vi "VALEW_ATC_Get ATC Data.vi"(0 "GEA2 Reference In":refnum<k24>, 11 "Error In":errorcluster) -> (4 "GEA2 Reference Out":refnum<k24>, 8 "ATC Data":T1, 15 "Error Out":errorcluster)   [LabVIEW 2016, in "TLMB.lvlib"]
uses:
  Projects/TLMB.lvlib
  typedefs/VALEW_ATC_Data.ctl
  Q:/Common/DLLs/GEA3/GeaCommunication.dll
  Common/DLLs/GEA3/GeaCommunication.dll
  Common/LabVIEW GEA2 Toolkit/LabVIEW_GEA2_Toolkit.lvlibp/type defs/ERD Read Data In.ctl
  Common/LabVIEW GEA2 Toolkit/LabVIEW_GEA2_Toolkit.lvlibp/type defs/Data Type.ctl
  Common/LabVIEW GEA2 Toolkit/LabVIEW_GEA2_Toolkit.lvlibp/type defs/Source_Destination.ctl
  Common/LabVIEW GEA2 Toolkit/LabVIEW_GEA2_Toolkit.lvlibp
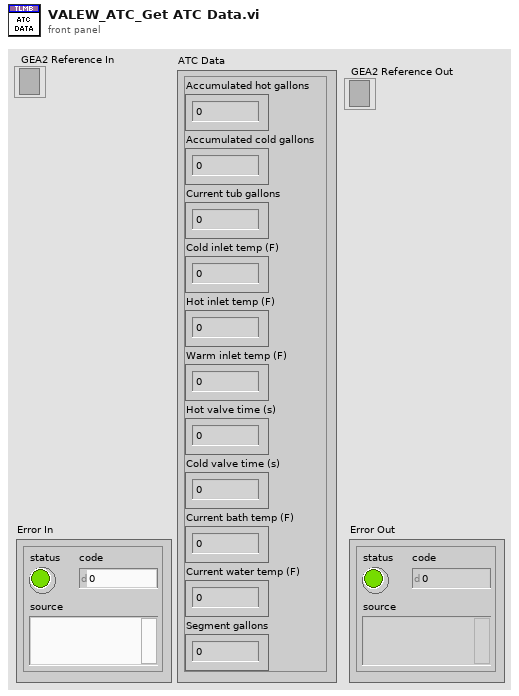
[diagram p1: front panel]
types:
  T1 = typedef "TLMB.lvlib/VALEW_ATC_Data.ctl" = cluster{"Accumulated hot gallons":dbl, "Accumulated cold gallons":dbl, "Current tub gallons":dbl, "Cold inlet temp (F)":dbl, "Hot inlet temp (F)":dbl, "Warm inlet temp (F)":dbl, "Hot valve time (s)":u16, "Cold valve time (s)":u16, "Current bath temp (F)":dbl, "Current water temp (F)":dbl, "Segment gallons":dbl}
  T2 = typedef "LabVIEW_GEA2_Toolkit.lvlibp/Source_Destination.ctl" = cluster{"Source":u8, "Destination":u8}
  T3 = typedef "LabVIEW_GEA2_Toolkit.lvlibp/ERD Read Data In.ctl" = cluster{"ERD Number":u16, "Data Type":T4}
  T4 = typedef "LabVIEW_GEA2_Toolkit.lvlibp/Data Type.ctl" = enum16{"string", "boolean", "uint8_t", "uint16_t", "uint32_t", "uint64_t", "int8_t", "int16_t", "int32_t", "int64_t"}
  T5 = typedef "LabVIEW_GEA2_Toolkit.lvlibp/ERD Read Data Out.ctl" = cluster{"ERD Number":u16, "Data":string}
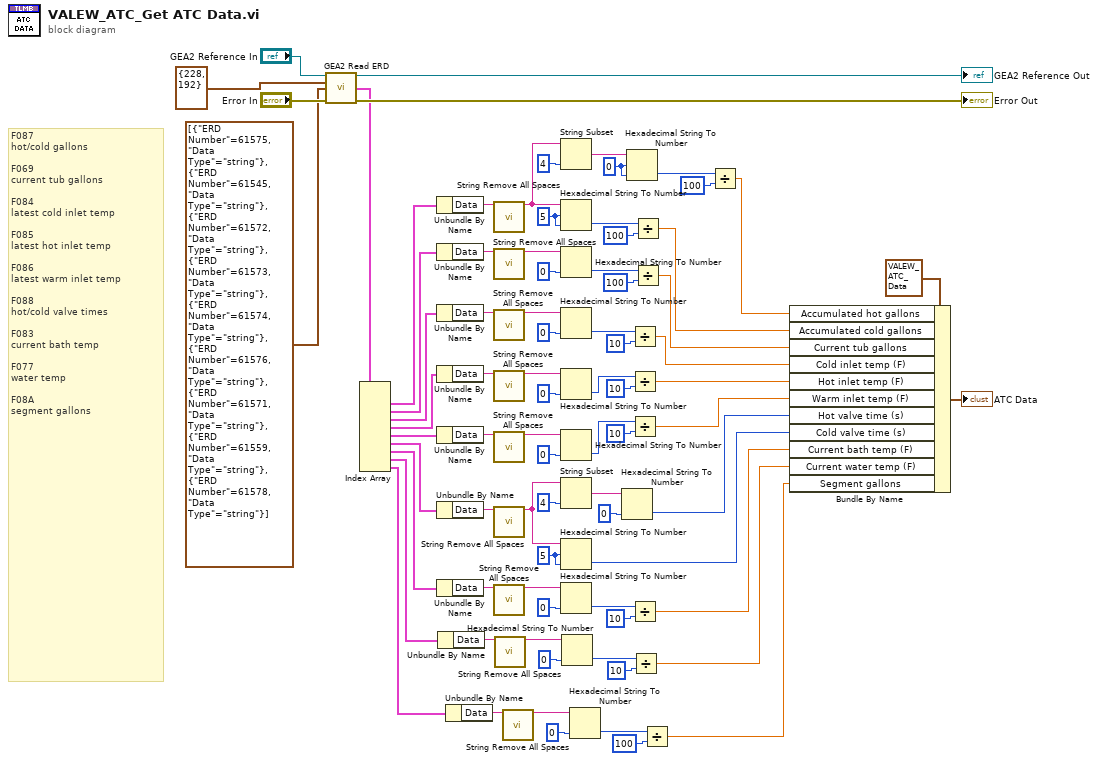
[diagram p0: block diagram]
diagram:
  w45 = u16 5 ("default (0 U32)")
  w75 = u16 0 ("default (0 U32)")
  w76 = u16 5 ("offset")
  # "F087\nhot/cold gallons\n\nF069\ncurrent tub gallons\n\nF084\nlatest cold inlet temp\n\nF085\nlatest hot inlet temp\n\nF086\nlatest warm inlet temp\n\nF088\nhot/cold valve times\n\nF083\ncurrent bath temp\n\nF077\nwater temp\n\nF08A\nsegment gallons"
  n1 = call "GEA2 Read ERD.vi"("GEA2 Reference In"="GEA2 Reference In", "GEA Inputs"=T2 {"Source"=228, "Destination"=192}, "Read ERD List"=T3[] [{"ERD Number"=61575, "Data Type"=enum."string"}, {"ERD Number"=61545, "Data Type"=enum."string"}, {"ERD Number"=61572, "Data Type"=enum."string"}, {"ERD Number"=61573, "Data Type"=enum."string"}, {"ERD Number"=61574, "Data Type"=enum."string"}, {"ERD Number"=61576, "Data Type"=enum."string"}, {"ERD Number"=61571, "Data Type"=enum."string"}, {"ERD Number"=61559, "Data Type"=enum."string"}, {"ERD Number"=61578, "Data Type"=enum."string"}], "Error In"="Error In") -> ("GEA2 Reference Out"=→"GEA2 Reference Out":refnum<k24>, "ERD Data Out"=w4:T5[], "Error Out"=→"Error Out":errorcluster)  [unwired: 8 in, 1 out]
  n2 = Index Array(array=w4) -> (element #1=w80:T5, element #2=w79:T5, element #3=w78:T5, element #4=w77:T5, element #5=w57:T5, element #6=w46:T5, element #7=w39:T5, element #8=w16:T5, element #9=w9:T5)  [unwired: 9 in]
  n3 = Unbundle By Name(w80) -> ("Data"=w61:string)
  n4 = Unbundle By Name(w79) -> ("Data"=w49:string)
  n5 = Unbundle By Name(w78) -> ("Data"=w52:string)
  n6 = Unbundle By Name(w77) -> ("Data"=w53:string)
  n7 = Unbundle By Name(w57) -> ("Data"=w56:string)
  n8 = Unbundle By Name(w46) -> ("Data"=w48:string)
  n9 = Unbundle By Name(w39) -> ("Data"=w43:string)
  n10 = Unbundle By Name(w16) -> ("Data"=w18:string)
  n11 = Unbundle By Name(w9) -> ("Data"=w14:string)
  n12 = call "String Remove All Spaces.vi"("Input String"=w61) -> ("Spaces Removed"=w27:string)  [unwired: 13 in, 1 out]
  n13 = call "String Remove All Spaces.vi"("Input String"=w49) -> ("Spaces Removed"=w50:string)  [unwired: 13 in, 1 out]
  n14 = call "String Remove All Spaces.vi"("Input String"=w52) -> ("Spaces Removed"=w51:string)  [unwired: 13 in, 1 out]
  n15 = call "String Remove All Spaces.vi"("Input String"=w53) -> ("Spaces Removed"=w54:string)  [unwired: 13 in, 1 out]
  n16 = call "String Remove All Spaces.vi"("Input String"=w56) -> ("Spaces Removed"=w55:string)  [unwired: 13 in, 1 out]
  n17 = call "String Remove All Spaces.vi"("Input String"=w48) -> ("Spaces Removed"=w22:string)  [unwired: 13 in, 1 out]
  n18 = call "String Remove All Spaces.vi"("Input String"=w43) -> ("Spaces Removed"=w44:string)  [unwired: 13 in, 1 out]
  n19 = call "String Remove All Spaces.vi"("Input String"=w18) -> ("Spaces Removed"=w17:string)  [unwired: 13 in, 1 out]
  n20 = call "String Remove All Spaces.vi"("Input String"=w14) -> ("Spaces Removed"=w13:string)  [unwired: 13 in, 1 out]
  n21 = String Subset(string=w27, length (rest)=4 ("length (rest)")) -> (substring=w25:string)  [unwired: 1 in]
  n22 = Hexadecimal String To Number(string=w27, offset=w76, default (0uL)=w76) -> (number=w71:u16)  [unwired: 1 out]
  n23 = Hexadecimal String To Number(string=w50, default (0uL)=u16 0 ("default (0 U32)")) -> (number=w68:u16)  [unwired: 1 in, 1 out]
  n24 = Hexadecimal String To Number(string=w51, default (0uL)=u16 0 ("default (0 U32)")) -> (number=w67:u16)  [unwired: 1 in, 1 out]
  n25 = Hexadecimal String To Number(string=w54, default (0uL)=u16 0 ("default (0 U32)")) -> (number=w62:u16)  [unwired: 1 in, 1 out]
  n26 = Hexadecimal String To Number(string=w55, default (0uL)=u16 0 ("default (0 U32)")) -> (number=w60:u16)  [unwired: 1 in, 1 out]
  n27 = String Subset(string=w22, length (rest)=4 ("length (rest)")) -> (substring=w23:string)  [unwired: 1 in]
  n28 = Hexadecimal String To Number(string=w22, offset=w45, default (0uL)=w45) -> (number=w30:u16)  [unwired: 1 out]
  n29 = Hexadecimal String To Number(string=w44, default (0uL)=u16 0 ("default (0 U32)")) -> (number=w40:u16)  [unwired: 1 in, 1 out]
  n30 = Hexadecimal String To Number(string=w17, default (0uL)=u16 0 ("default (0 U32)")) -> (number=w21:u16)  [unwired: 1 in, 1 out]
  n31 = Hexadecimal String To Number(string=w13, default (0uL)=u16 0 ("default (0 U32)")) -> (number=w12:u16)  [unwired: 1 in, 1 out]
  n32 = Hexadecimal String To Number(string=w23, default (0uL)=u16 0 ("default (0 U32)")) -> (number=w31:u16)  [unwired: 1 in, 1 out]
  n33 = Hexadecimal String To Number(string=w25, offset=w75, default (0uL)=w75) -> (number=w74:u16)  [unwired: 1 out]
  n34 = Divide(x=w67, y=u16 10) -> (x/y=w34:dbl)
  n35 = Divide(x=w62, y=u16 10) -> (x/y=w33:dbl)
  n36 = Divide(x=w60, y=u16 10) -> (x/y=w32:dbl)
  n37 = Divide(x=w40, y=u16 10) -> (x/y=w29:dbl)
  n38 = Divide(x=w21, y=u16 10) -> (x/y=w15:dbl)
  n39 = Divide(x=w71, y=u16 100) -> (x/y=w36:dbl)
  n40 = Divide(x=w68, y=u16 100) -> (x/y=w35:dbl)
  n41 = Divide(x=w12, y=u16 100) -> (x/y=w8:dbl)
  n42 = Divide(x=w74, y=u16 100) -> (x/y=w37:dbl)
  n43 = Bundle By Name(cluster=T1 {"Accumulated hot gallons"=0.0, "Accumulated cold gallons"=0.0, "Current tub gallons"=0.0, "Cold inlet temp (F)"=0.0, "Hot inlet temp (F)"=0.0, "Warm inlet temp (F)"=0.0, "Hot valve time (s)"=0, "Cold valve time (s)"=0, "Current bath temp (F)"=0.0, "Current water temp (F)"=0.0, "Segment gallons"=0.0} ("ATC Data 2"), "Accumulated hot gallons"=w37, "Accumulated cold gallons"=w36, "Current tub gallons"=w35, "Cold inlet temp (F)"=w34, "Hot inlet temp (F)"=w33, "Warm inlet temp (F)"=w32, "Hot valve time (s)"=w31, "Cold valve time (s)"=w30, "Current bath temp (F)"=w29, "Current water temp (F)"=w15, "Segment gallons"=w8) -> (→"ATC Data":T1)
